vi "climber.vi"(11 "compressorDev":T1) -> (3 "motorSpeed":dbl)   [LabVIEW 2016]
uses:
  <vilib>/Rock Robotics/WPI/Compressor/WPI_CompressorDevRef.ctl
  <vilib>/Rock Robotics/WPI/Utilities/WPI_GetSetVariantRefNum.vi
  Robot Global Data.vi
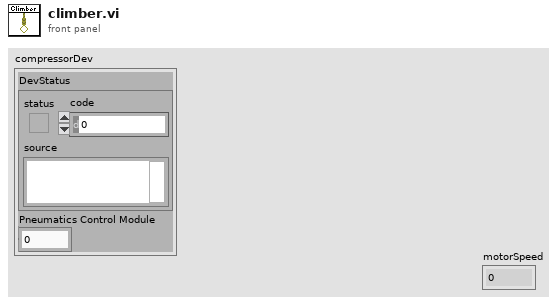
[diagram p1: front panel]
types:
  T1 = typedef "WPI_CompressorDevRef.ctl" = cluster{"DevStatus":errorcluster, "Pneumatics Control Module":u8}
  T2 = typedef "WPI_JoystickDevRef.ctl" = cluster{"Device":T3}
  T3 = typedef "WPI_JoystickDeviceEnum.ctl" = enum16{"USB 0", "USB 1", "USB 2", "USB 3", "USB 4", "USB 5"}
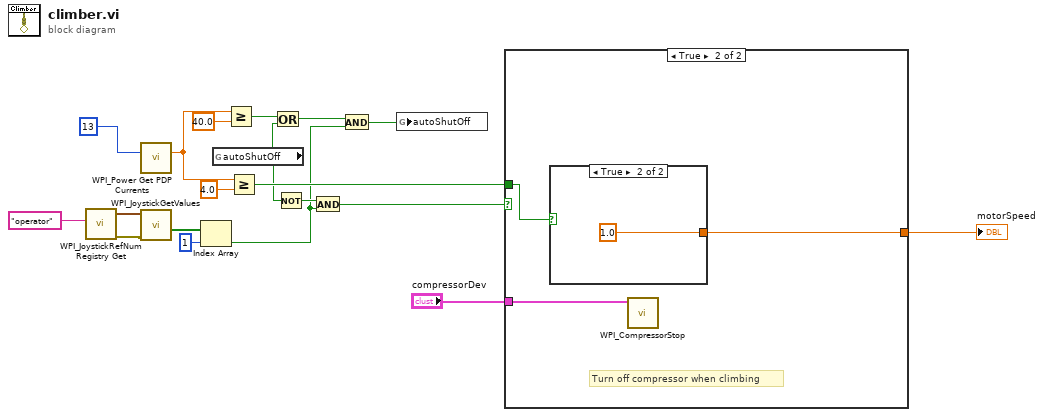
[diagram p0: block diagram]
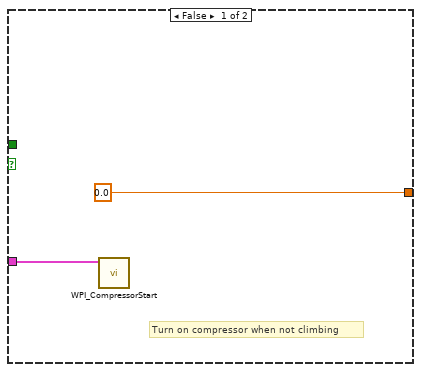
[diagram p2: hidden frame]
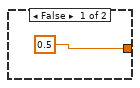
[diagram p3: hidden frame]
diagram:
  n1 = call <vilib>:"WPI_JoystickRefNum Registry Get.vi"("refnum name"="operator") -> ("error out"=w16:errorcluster, "JoystickDevRef"=w17:T2)  [unwired: 9 in]
  n2 = call <vilib>:"WPI_Power Get PDP Currents.vi"("PDP Channel"=13) -> ("current (A)"=w9:dbl)  [unwired: 12 in, 2 out]
  n3 = call <vilib>:"WPI_JoystickGetValues.vi"("error in (no error)"=w16, "JoystickDevRef"=w17) -> ("Buttons"=w18:bool[])  [unwired: 5 in, 4 out]
  n4 = Index Array(array=w18, index=1) -> (element=w1:bool)
  n5 = global read "Robot Global Data.vi" "autoShutOff"() -> (w5:bool)
  n6 = Greater Or Equal?(x=w9, y=40.0) -> (x >= y?=w6:bool)
  n7 = Greater Or Equal?(x=w9, y=4.0) -> (x >= y?=w7:bool)
  n8 = Or(x=w6, y=w5) -> (x .or. y?=w2:bool)
  n9 = Not(x=w5) -> (.not. x?=w4:bool)
  n10 = And(x=w4, y=w1) -> (x .and. y?=w10:bool)
  n11 = And(x=w2, y=w1) -> (x .and. y?=w3:bool)
  n12 = global write "Robot Global Data.vi" "autoShutOff"(w3) -> ()
  n13 = case shown="True" w10 {
    tunnel: [0.0 w24] -> w14
    tunnel: "compressorDev" -> [w20 w23]
    tunnel: w7 -> [_ w22]
    frame False {
      # "Turn on compressor when not climbing"
      n14 = call <vilib>:"WPI_CompressorStart.vi"("CompressorDevRef"=w20) -> ()  [unwired: 9 in, 2 out]
    }
    frame True {
      # "Turn off compressor when climbing"
      n15 = case shown="True" w22 {
        tunnel: [0.5 1.0] -> w24
        frame False {
        }
        frame True {
        }
      }
      n16 = call <vilib>:"WPI_CompressorStop.vi"("CompressorDevRef"=w23) -> ()  [unwired: 9 in, 2 out]
    }
  }
  "motorSpeed" <- w14
